vi "Angle_M.vi"() -> ()   [LabVIEW 2024]
panel:
  in  "Path":path
  out "return value":dbl
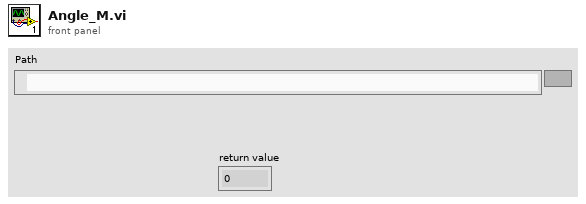
[diagram p1: front panel]
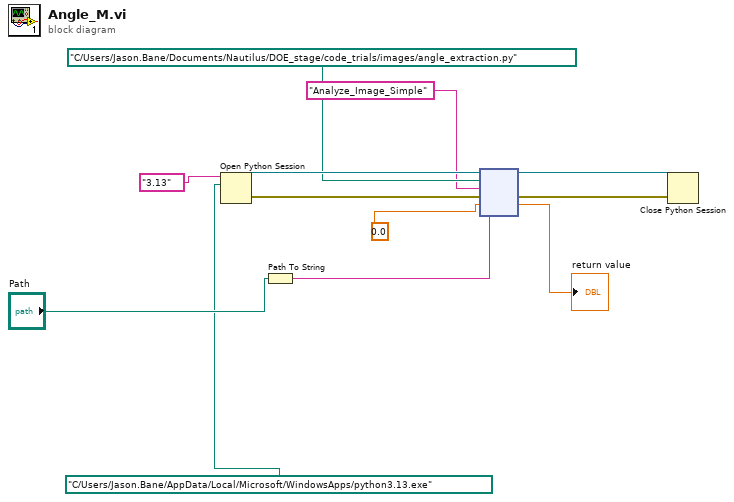
[diagram p0: block diagram]
diagram:
  n1 = Open Python Session(python version="3.13" ("Python version"), python path=path "C:/Users/Jason.Bane/AppData/Local/Microsoft/WindowsApps/python3.13.exe" ("Python path")) -> (session out=w11:refnum<k35>, error out=w9:errorcluster)  [unwired: 1 in]
  n2 = Path To String(path="Path") -> (string=w3:string)
  n3 = node(w11, path "C:/Users/Jason.Bane/Documents/Nautilus/DOE_stage/code_trials/images/angle_extraction.py" ("module path"), "Analyze_Image_Simple" ("function name"), w9, 0.0 ("return type"), w3) -> (w10:refnum<k35>, w8:errorcluster, →"return value":dbl)  [unwired: 1 in, 2 out]
  n4 = Close Python Session(session in=w10, error in=w8) -> ()  [unwired: 1 out]
